vi "UpdateSystemParams_SM.vi"(8 "error in (no error)":errorcluster, 10 "Override File Path":path=path "C:/Users/veenaj/Desktop/ZenGage V1.2.2/Configuration file/Zengage System JSON Override.json", 11 "Cluster In":T2) -> (0 "error out":errorcluster, 3 "Cluster Out":T2)   [LabVIEW 2019, in "Inspection Statemachine.lvclass"]
uses:
  Inspection Statemachine.lvclass
  <vilib>/vision/Image Controls.llb/IMAQ Image.ctl
  Controls/Result Cluster_SM.ctl
  Common/Controls/Pop-up Input.ctl
  Common/Controls/Camera Optics Diagnostics Result.ctl
  Common/Controls/AllPartInfo.ctl
  Controls/Output Cluster_SM.ctl
  Controls/LocalData_SM.ctl
panel:
  in  "Override":T1={"SystemParameters"={"SystemName"="", "SystemID"="", "SoftwareFeatures"={"DoorPokayokeEnable"=TRUE, "FailCountDisplayEnable"=FALSE, "FailCountReversalEnable"=FALSE}}}
  out "VCluster\n Override":variant
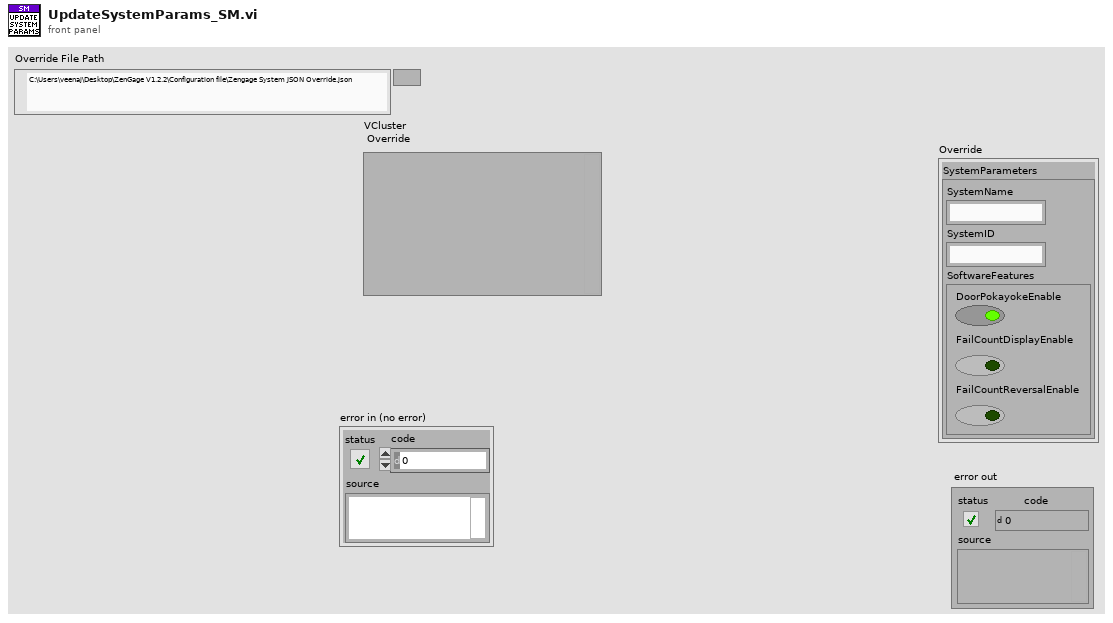
[diagram p1: front panel]
types:
  T1 = cluster{"SystemParameters":cluster{"SystemName":string, "SystemID":string, "SoftwareFeatures":cluster{"DoorPokayokeEnable":bool, "FailCountDisplayEnable":bool, "FailCountReversalEnable":bool}}}
  T2 = typedef "Inspection Statemachine.lvclass/LocalData_SM.ctl" = cluster{"Timeout":i32, "Core":cluster{"Current VI Reference":refnum<vi>, "Close Panel on Exit?":bool}, "Ack":u8, " CurrentState":string, "DirectExit":bool, "SoftwareExit":bool, "SensorDiagnosticsStatus":bool, "OutputCluster":T3, "SelComplete":bool, "ResultToMI":bool, "Exit":bool, "NumberOfActorsLaunched":i32, "BatchStart":bool, "LoadingBarActive":bool, "UpdateInPause":bool, " EventReason":string, "PopUpCategory":string, "PopUpActive":bool, "MasterSampleState":string, "CameraOpticsDiagnosticsStatus":bool, "CameraIndex":i32, "SensorIndex":i32}
  T3 = typedef "Inspection Statemachine.lvclass/Output Cluster_SM.ctl" = cluster{"RackID":u8, "Trigger Light Camera Sequence":cluster{"Light Sequence Trigger":string, "Status":string, "Mode":string}, "Result Cluster":T4, "Analytics VI refnum":refnum<vi>, "Statistical parameters ":string[][], "Sensor Name":string, "Camera Name":string, "PopupInput":T6, "PartInfo":cluster{"PartName":string, "NumberOfRacks":u8, "TotalCount":u64, "ReelCount":u64, "OperatorName":string, "StampingMachineID":u32, "RackID":u8, "Reinitialize":bool, "MeasurementNamesArray":string[], "MeasurementIDArray":u16[], "SpecValuesArray":cluster{"LCL":dbl, "UCL":dbl, "LSL":dbl, "USL":dbl, "Nominal Value":dbl}[], "CameraNamesArray":string[]}, "StateMsgToMI":string, "InspectionStatusToMI":string, "StateMsgToRC":string, "StateMsgToUI":string, "StateMsgToDL":string, "StateMsgToAN":string, "StateMsgToSM":string, "EventData":cluster{"EventName":string, "EventReason":string}, "CameraOpticsDiagnosticsResult":T7, "AllPartInfo":T8, "SystemParameters":cluster{"SystemName":string, "SystemID":string, "CustomerDetails":cluster{"CustomerName":string, "CustomerId":string, "Location":string, "NumberOfShifts":dbl, "ShiftDetails":cluster{"Name":string, "Timing":string}[]}, "InstallationDate":string, "NextServiceDate":string, "NumberOfRacks":u8, "TotalNumberOfCameras":u8, "SoftwareFeatures":cluster{"HardwareEmulated":bool, "PowerOnSelfTest":bool, "DiagnosticsEnable":bool, "AnalyticsEnable":bool, "DefectTrackingEnable":bool, "AutomaticGuideMovement":bool, "DoorPokayokeEnable":bool, "FailCountDisplayEnable":bool, "FailCountReversalEnable":bool, "DataLoggingEnable":bool, "PauseOnReelCountFinish":bool, "StopOnTotalCountFinish":bool, "IoTEnable":bool, "ReportEnable":bool, "DebugLevel":dbl, "PowerOnSelfTestFeatures":cluster{"TimingUnit":bool, "MachinePowerStatusCheck":bool, "GuideMotor":bool, "CameraOptics":bool, "MasterSample":bool}, "DiagnosticsFeatures":cluster{"TimingUnit":bool, "GuideMotor":bool, "CameraOptics":bool, "ReelerMotor":bool, "HardwareButtons":bool, "Sensors":bool, "TowerLamp":bool, "MasterSample":bool}, "UserInterface":cluster{"DynamicImageHandlingEnable":bool, "DoorPokaYokeButtonVisible":bool, "FailCountDisplayButtonVisible":bool, "FailCountReversalButtonVisible":bool}, "PopupOptions":cluster{"ReasonForPause":bool, "ReasonForFail":bool, "ReasonForStop":bool, "CpCpkOnReelFinish":bool}, "DataloggingFeatures":cluster{"EventData":bool, "MeasurementData":bool, "StatisticalData":bool, "ReelData":bool, "FailedMeasurementData":bool, "FailedImages":bool}, "IoT":cluster{"SMSAlertEnable":bool, "EmailAlertEnable":bool}}}, "PartsConfigured":cluster{"Name":string, "NumberOfRack":u8}[], "CameraSequenceList":cluster{"Name":string, "RackID":u8}[], "SensorList":cluster{"Name":string, "RackID":u8}[], "MasterSampleMessages":cluster{"MasterSampleMessage":string, "PartMessage":string}, "SensorDiagnosticsResult":cluster{"Image Array":T5[], "ImageCount":u64}, "IgnoredCountDetails":cluster{"ReelCount":u64, "TotalCount":u64}, "MachineStatusToDL":string, "MasterSamplePartName":string}
  T4 = typedef "Inspection Statemachine.lvclass/Result Cluster_SM.ctl" = cluster{"RackID":u8, "MeasurementValuesArray ":dbl[], "ImagesArray":T5[], "ResultPF":bool, "ProductionCountDetails":cluster{"TotalFail":u64, "TotalPass":u64, "TotalCount":u64}, "ReelCountDetails":cluster{"ReelFail":u64, "ReelPass":u64, "ReelCount":u64}, "ControlPFArray":bool[], "SpecificationPFArray":bool[], "SpecificationFail":bool, "ReelNumber":u64, "Status":string}
  T5 = typedef "IMAQ Image.ctl" = refnum<image>
  T6 = typedef "Pop-up Input.ctl" = cluster{"Pop-up Type":enum16{"Open Logo Display", "Close Logo Display", "Open Loading Bar", "Close Loading Bar", "Open Alert Display", "Close Alert Display", "One button dialog box", "Two button dialog box", "User Authentication"}, "Title":string, "Message":string, "Button 1 Text":string, "Button 2 Text":string, "Show Close? T/F":bool, "Title Blink? T/F":bool, "Title Blink Colour":u32}
  T7 = typedef "Camera Optics Diagnostics Result.ctl" = cluster{"LightCameraName":string, "DiagnosedImage":T5, "DustPercentage":dbl, "Result":bool}
  T8 = typedef "AllPartInfo.ctl" = cluster{"PartName":string, "NumberOfRacks":u8, "MeasurementIDsArray":u16[], "MeasurementNamesArray":string[], "SpecValuesArray":cluster{"LCL":dbl, "UCL":dbl, "LSL":dbl, "USL":dbl, "NominalValue":dbl}[]}[]
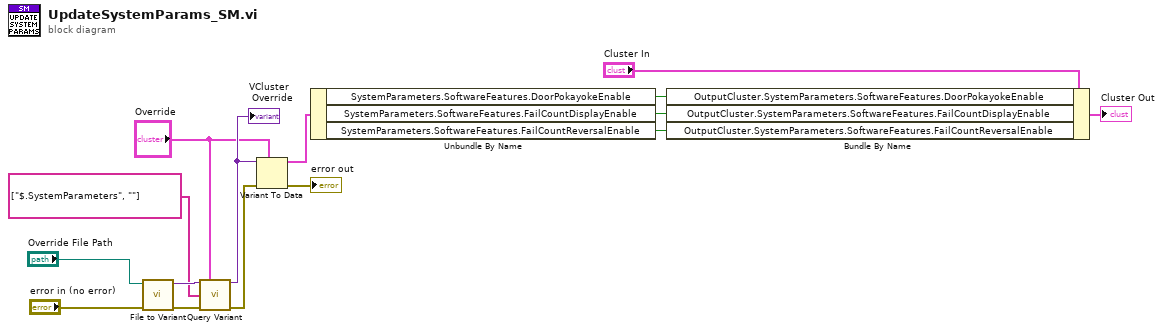
[diagram p0: block diagram]
diagram:
  n1 = call <vilib>:"File to Variant.vi"("JSON FilePath"="Override File Path", "error in (no error)"="error in (no error)") -> ("JSON Variant"=w13:variant, "error out"=w12:errorcluster)  [unwired: 6 in, 1 out]
  n2 = call <vilib>:"Query Variant.vi"("VCluster in"=w13, "Reference Variant"="Override", "pathList"=string[] ["$.SystemParameters", ""], "error IO"=w12) -> ("VCluster\n out"=w10:variant, "error out"=w9:errorcluster)  [unwired: 8 in, 2 out]
  "VCluster\n Override" <- w10
  n3 = Variant To Data(error in=w9, type="Override", Variant=w10) -> (data=w8:T1, error out=→"error out":errorcluster)
  n4 = Unbundle By Name(w8) -> ("SystemParameters.SoftwareFeatures.DoorPokayokeEnable"=w7:bool, "SystemParameters.SoftwareFeatures.FailCountDisplayEnable"=w2:bool, "SystemParameters.SoftwareFeatures.FailCountReversalEnable"=w1:bool)
  n5 = Bundle By Name(cluster="Cluster In", "OutputCluster.SystemParameters.SoftwareFeatures.DoorPokayokeEnable"=w7, "OutputCluster.SystemParameters.SoftwareFeatures.FailCountDisplayEnable"=w2, "OutputCluster.SystemParameters.SoftwareFeatures.FailCountReversalEnable"=w1) -> (→"Cluster Out":T2)
